vi "Endpoint Connected.vi"(8 "error in":errorcluster, 10 "Endpoint":refnum<class "Message Enqueuer.lvclass">, 11 "MSS Target Actor in":refnum<class "MSS Target Actor.lvclass">) -> (0 "error out":errorcluster, 3 "MSS Target Actor out":refnum<class "MSS Target Actor.lvclass">)   [LabVIEW 2023, in "MSS Target Actor.lvlib" / "MSS Target Actor.lvclass"]
doc: "Override this method to specify how the receiving actor responds to a Connected message from a nested endpoint actor."
uses:
  MSS Target Actor.lvclass
  <vilib>/ActorFramework/Message Enqueuer/Message Enqueuer.lvclass
  MSS Target Actor.lvclass/MSS Target Actor.ctl
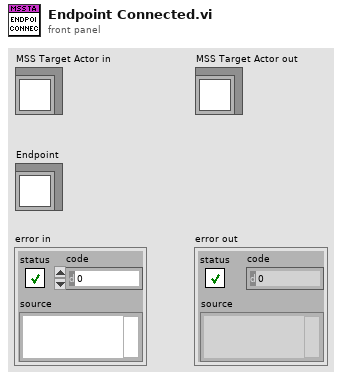
[diagram p1: front panel]
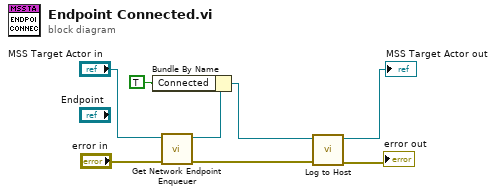
[diagram p0: block diagram]
diagram:
  n1 = call "Get Network Endpoint Enqueuer.vi"("error in"="error in", "MSS Target Actor in"="MSS Target Actor in") -> ("error out"=w7:errorcluster, "MSS Target Actor out"=w3:refnum<class "MSS Target Actor.lvclass">)  [unwired: 6 in, 2 out]
  n2 = Bundle By Name(cluster=w3, "Connected"=TRUE) -> (w2:refnum<class "MSS Target Actor.lvclass">)
  n3 = call "Log to Host.vi"("error in"=w7, "MSS Target Actor in"=w2) -> ("error out"=→"error out":errorcluster, "MSS Target Actor out"=→"MSS Target Actor out":refnum<class "MSS Target Actor.lvclass">)  [unwired: 8 in]
